vi "FFT Spectrum (Mag-Phase) for N Chan (CDB).vi"(4 "window parameter":dbl=nan, 6 "averaging parameters":T2={"averaging mode"=enum."No averaging", "weighting mode"=enum."Exponential", "number of averages"=10} {"number of averages" min=1}, 7 "restart averaging (F)":bool, 8 "error in (no error)":errorcluster, 9 "view":T1, 10 "window":T3=1 items=["Rectangle"=0, "Hanning"=1, "Hamming"=2, "Blackman-Harris"=3, "Exact Blackman"=4, "Blackman"=5, "Flat Top"=6, "4 Term B-Harris "=7, "7 Term B-Harris"=8, "Low Sidelobe"=9, "Blackman Nuttall"=11, "Triangle"=30, "Bartlett-Hanning"=31, "Bohman"=32, "Parzen"=33, "Welch"=34, "Kaiser"=60, "Dolph-Chebyshev"=61, "Gaussian"=62], 11 "time signals":waveform(cdb)[](array[waveform])) -> (0 "error out":errorcluster, 1 "averages completed":dbl, 2 "phases":cluster{"f0":dbl, "df":dbl, "phase":dbl[]}[](array[cluster]) {"phase" format="%.2p"; "f0" format="%.2p"; "df" format="%.2p"}, 3 "magnitudes":cluster{"f0":dbl, "df":dbl, "magnitude":dbl[]}[](array[cluster]) {"magnitude" format="%.2p"; "f0" format="%.2p"; "df" format="%.2p"}, 5 "averaging done":bool)   [LabVIEW 2020, in "NI_MAPro.lvlib"]
doc: "Computes the averaged FFT spectrum of <B>time signal</B>. This VI returns the FFT results as <B>magnitude</B> and <B>phase</B>. Wire data to the <B>time signal</B> input to determine the polymorphic instance to use or manually select the instance."
uses:
  NI_MAPro.lvlib
  windowTd.ctl
  NI_MABase.lvlib
  NI_AALPro.lvlib
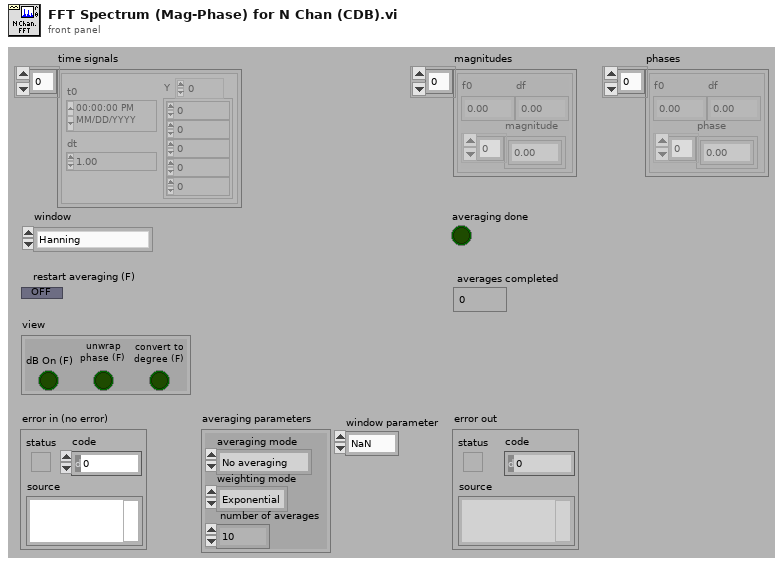
[diagram p1: front panel]
types:
  T1 = cluster{"dB On (F)":bool, "unwrap phase (F)":bool, "convert to degree (F)":bool}
  T2 = cluster{"averaging mode":enum16{"No averaging", "Vector averaging", "RMS averaging", "Peak hold"}, "weighting mode":enum16{"Linear", "Exponential"}, "number of averages":u32}
  T3 = typedef "NI_AALPro.lvlib/windowTd.ctl" = u32
  T4 = cluster{"block size":i32, "dt":dbl, "spectrum parameters":cluster{"averaging parameters":cluster{"averaging mode":enum16{"No averaging", "Vector averaging", "RMS averaging", "Peak hold"}, "weighting mode":enum16{"Linear", "Exponential"}, "number of averages":u32}, "window":T3}, "df":dbl, "averages completed":dbl, "complex spectrum":cdb[], "real spectrum":dbl[], "t0 history":dbl, "dt history":dbl, "timestamp":dbl, "lin avg done":bool}
  T5 = cluster{"f0":dbl, "df":dbl, "imag or phase":dbl[]}
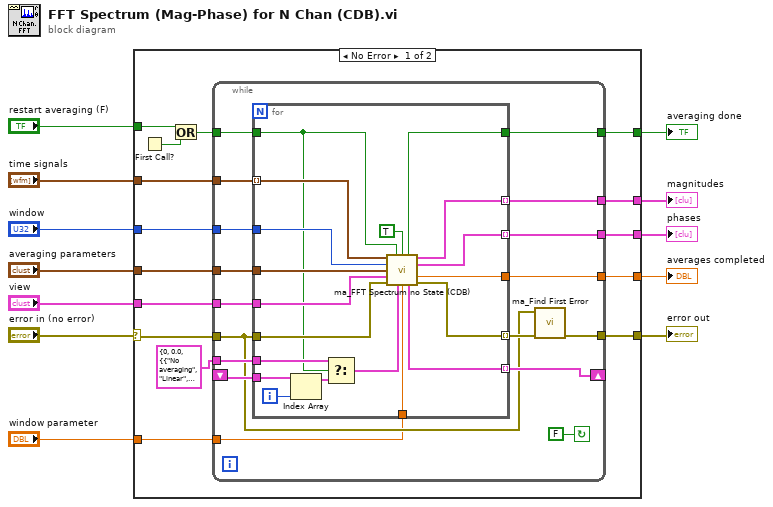
[diagram p0: block diagram]
diagram:
  n1 = case shown="No Error" "error in (no error)" {
    selector: "error in (no error)" -> [w25 w64]
    tunnel: [w23 w64] -> w12
    tunnel: "restart averaging (F)" -> [w22 _]
    tunnel: "time signals" -> [w21 _]
    tunnel: "window" -> [w20 _]
    tunnel: "averaging parameters" -> [w19 _]
    tunnel: "view" -> [w18 _]
    tunnel: "window parameter" -> [w17 _]
    tunnel: [w16 _] -> w4
    tunnel: [w15 _] -> w3
    tunnel: [w14 _] -> w2
    tunnel: [w13 _] -> w1
    frame No Error {
      n2 = First Call?() -> (First Call?: T/F=w27:bool)
      n3 = Or(x=w22, y=w27) -> (x .or. y?=w26:bool)
      n4 = while {
        tunnel: [w44] -> w16
        tunnel: [w43] -> w13
        tunnel: [w42] -> w15
        tunnel: [w30] -> w23
        shift-right: [w40] -> _
        shift-left: _ -> [w39]
        tunnel: w26 -> [w37]
        tunnel: w21 -> [w36]
        tunnel: w20 -> [w35]
        tunnel: w19 -> [w34]
        tunnel: w18 -> [w33]
        tunnel: w25 -> [w29]
        tunnel: [w32] -> w14
        tunnel: T4 {"block size"=0, "dt"=0.0, "spectrum parameters"={"averaging parameters"={"averaging mode"=enum."No averaging", "weighting mode"=enum."Linear", "number of averages"=0}, "window"=0}, "df"=0.0, "averages completed"=0.0, "complex spectrum"=[], "real spectrum"=[], "t0 history"=0.0, "dt history"=0.0, "timestamp"=0.0, "lin avg done"=FALSE} ("state info") -> [w31]
        tunnel: w17 -> [w28]
        stop <- FALSE continue-if-true
        n5 = for {
          tunnel: [w63] -> w44
          tunnel: [w62] -> w43
          tunnel: [w61] -> w42 mode=indexing
          tunnel: [w60] -> w41 mode=indexing
          tunnel: [w59] -> w40 mode=indexing
          tunnel: w39 -> [w57]
          tunnel: w37 -> [w46]
          tunnel: w36 -> [w53] mode=indexing
          tunnel: w35 -> [w52]
          tunnel: w34 -> [w51]
          tunnel: w33 -> [w50]
          tunnel: w29 -> [w49]
          tunnel: [w48] -> w32 mode=indexing
          tunnel: w31 -> [w47]
          tunnel: w28 -> [w45]
          i -> [w56]
          n6 = Index Array(array=w57, index=w56) -> (element=w55:T4)
          n7 = Select(t=w47, s=w46, f=w55) -> (s? t:f=w58:T4)
          n8 = call "ma_FFT Spectrum no State (CDB).vi"("time signal"=w53, "restart averaging (F)"=w46, "mag-phase"=TRUE, "window"=w52, "averaging parameters"=w51, "view"=w50, "error in"=w49, "state info"=w58, "window parameter"=w45) -> ("averaging done"=w63:bool, "real or mag"=w61:cluster{"f0":dbl, "df":dbl, "real or mag":dbl[]}, "imag or phase"=w48:T5, "averages completed"=w62:dbl, "state info"=w59:T4, "error out"=w60:errorcluster)  [unwired: 1 out]
        }
        n9 = call "ma_Find First Error.vi"("error array in"=w41, "error in 1 (no error)"=w29) -> ("error out"=w30:errorcluster)  [unwired: 2 in, 3 out]
      }
    }
    frame Error {
    }
  }
  "error out" <- w12
  "averages completed" <- w1
  "averaging done" <- w4
  "phases" <- w2
  "magnitudes" <- w3
